vi "I32ArrayToStr(cast).vi"(1 "I64数组":i64[](array[numeric]) format="%.0x") -> (0 "字符串":string)   [LabVIEW 2012]
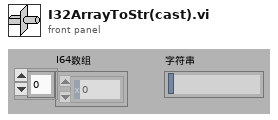
[diagram p1: front panel]
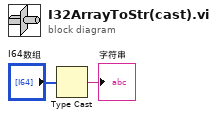
[diagram p0: block diagram]
diagram:
  n1 = Type Cast(x="I64数组") -> (*(type *) &x=→"字符串":string)  [unwired: 1 in]
